vi "sub_writeGuessToDebugString.vi"(9 "guess":T1) -> ()   [LabVIEW 2018]
uses:
  guess.ctl
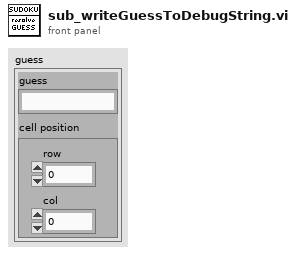
[diagram p1: front panel]
types:
  T1 = typedef "guess.ctl" = cluster{"cell position":cluster{"row":i32, "col":i32}, "guess":string}
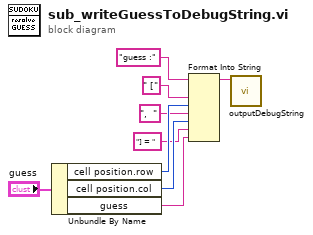
[diagram p0: block diagram]
diagram:
  n1 = Unbundle By Name("guess") -> ("cell position.row"=w8:i32, "cell position.col"=w7:i32, "guess"=w1:string)
  n2 = Format Into String(initial string="guess :", " [", w8, ",  ", w7, "] = ", w1) -> (resulting string=w2:string)  [unwired: 2 in, 1 out]
  n3 = call "outputDebugString.vi"("arg1"=w2) -> ()  [unwired: 11 in]
